vi "Vehicle Control.vi"(11 "stop":bool) -> ()   [LabVIEW 2012]
uses:
  Formula Hybrid 2012 r1/Global Data.vi
  <vilib>/FPGAPlugInAG/cRIO-9076/niLvFpga_Open_cRIO-9076.vi
  <vilib>/rvi/interface/common/dynamic/niFpgaDynamicAddResources.vi
  <vilib>/Utility/error.llb/Error Cluster From Error Code.vi
  <vilib>/rvi/errors/niLvFpgaAdjustHostInterfaceError.vi
  <vilib>/addons/control/pid/pid.llb/PID (DBL).vi
  <vilib>/rvi/interface/nirviOpenFPGA/nirviOpenFPGA.xnode
  FPGA Bitfiles/FormulaHybrid201_FPGATarget_FPGA_E9E2F20A.lvbitx
  Formula Hybrid 2012 r1/FPGA/Sensor Library/FPGA.vi
  <vilib>/rvi/interface/nirviReadWriteControl/nirviReadWriteControl.xnode
  <vilib>/rvi/interface/Simulation/niFpgaSimulationCallBeginRW.vi
  <vilib>/addons/control/pid/NI_PID_pid.lvlib
  NiFpgaLv.dll
panel:
  in  "Lateral PID gains":T1={"proportional gain (Kc)"=1.0, "integral time (Ti, min)"=0.01, "derivative time (Td, min)"=0.0} {"derivative time (Td, min)" format="%.3f"; "integral time (Ti, min)" format="%.3f"; "proportional gain (Kc)" format="%.3f"}
  in  "Allowable Variation from Ideal (Lateral)":dbl=0.1
  in  "Ideal Lateral Slip (%)":dbl=1.2
  out "Throttle Percent":fxp<+,14,1>
  in  "Inline PID gains":T1={"proportional gain (Kc)"=1.0, "integral time (Ti, min)"=0.01, "derivative time (Td, min)"=0.0} {"derivative time (Td, min)" format="%.3f"; "integral time (Ti, min)" format="%.3f"; "proportional gain (Kc)" format="%.3f"}
  in  "Allowable Variation from Ideal (Inline)":dbl=0.1
  in  "Ideal Inline Slip (%)":dbl=1.2
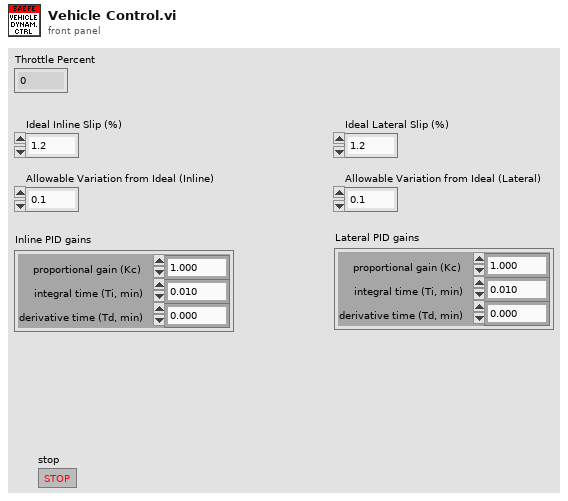
[diagram p1: front panel]
types:
  T1 = cluster{"proportional gain (Kc)":dbl, "integral time (Ti, min)":dbl, "derivative time (Td, min)":dbl}
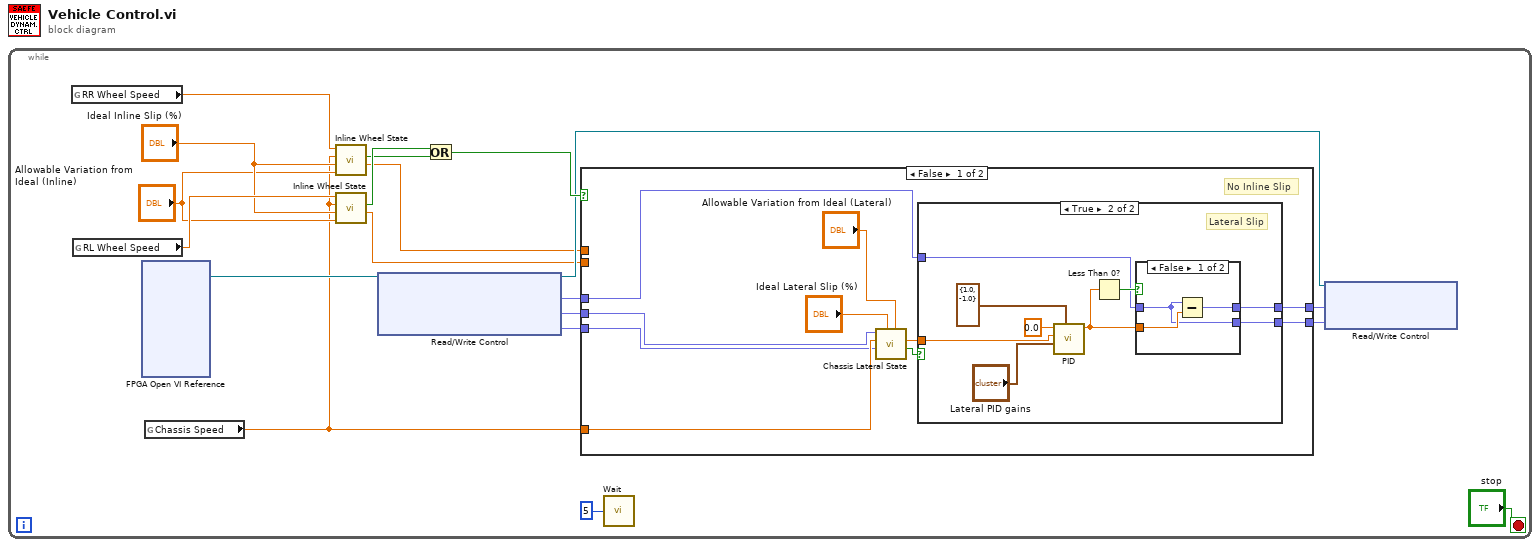
[diagram p0: block diagram]
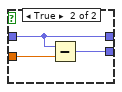
[diagram p3: hidden frame]
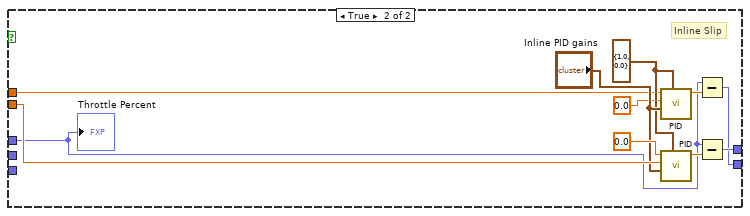
[diagram p4: hidden frame]
diagram:
  n1 = while {
    stop <- "stop" stop-if-true
    n2 = global read "Global Data.vi" "RR Wheel Speed"() -> (w14:dbl)
    n3 = global read "Global Data.vi" "RL Wheel Speed"() -> (w17:dbl)
    n4 = xnode "FPGA Open VI Reference"() -> ("FPGA VI Reference Out"=w10:refnum<k20>)  [unwired: 2 in, 1 out]
    n5 = global read "Global Data.vi" "Chassis Speed"() -> (w3:dbl)
    n6 = call "Inline Wheel State.vi"("Allowable Variation from Ideal"="Allowable Variation from Ideal (Inline)", "Ideal Slip Percent"="Ideal Inline Slip (%)", "Chassis Speed"=w3, "Wheel Speed"=w14) -> ("Error"=w4:dbl, "Inline Slip"=w11:bool)  [unwired: 6 in]
    n7 = call "Inline Wheel State.vi"("Allowable Variation from Ideal"="Allowable Variation from Ideal (Inline)", "Ideal Slip Percent"="Ideal Inline Slip (%)", "Chassis Speed"=w3, "Wheel Speed"=w17) -> ("Error"=w5:dbl, "Inline Slip"=w12:bool)  [unwired: 6 in]
    n8 = xnode "Read/Write Control"("FPGA VI Reference In"=w10) -> ("FPGA VI Reference Out"=w9:refnum<k20>, "Average Throttle (%)"=w8:fxp<+/-,29,18>, "Rotation Rate (degrees/s)"=w2:fxp<+/-,48,26>, "Steering Wheel Angle (degrees)"=w1:fxp<+/-,58,35>)  [unwired: 1 in, 1 out]
    n9 = Or(x=w12, y=w11) -> (x .or. y?=w13:bool)
    n10 = case shown="False" w13 {
      tunnel: w8 -> [w28 w46]
      tunnel: [w27 w53] -> w7
      tunnel: [w26 w47] -> w6
      tunnel: w5 -> [_ w56]
      tunnel: w4 -> [_ w50]
      tunnel: w3 -> [w24 _]
      tunnel: w2 -> [w23 _]
      tunnel: w1 -> [w22 _]
      frame False {
        # "No Inline Slip"
        n11 = call "Chassis Lateral State.vi"("Allowable Variation from Idea"="Allowable Variation from Ideal (Lateral)", "Ideal Lateral Slip"="Ideal Lateral Slip (%)", "Steering Angle"=w22, "Chassis Speed"=w24, "Chassis Yaw Rate"=w23) -> ("Lateral Slip"=w29:bool, "Error"=w25:dbl)  [unwired: 5 in]
        n12 = case shown="True" w29 {
          tunnel: w28 -> [w30 w34]
          tunnel: [w30 w32] -> w27
          tunnel: [w30 w33] -> w26
          tunnel: w25 -> [_ w39]
          frame False {
            # "No Lateral Slip"
          }
          frame True {
            # "Lateral Slip"
            n13 = call-poly <vilib>:"PID.vi"("output range"=cluster{"output high":dbl, "output low":dbl} {"output high"=1.0, "output low"=-1.0}, "PID gains"="Lateral PID gains", "process variable"=w39, "setpoint"=0.0) -> ("output"=w35:dbl)  [unwired: 6 in, 1 out]
            n14 = Less Than 0?(x=w35) -> (x < 0?=w36:bool)
            n15 = case shown="False" w36 {
              tunnel: w35 -> [w42 w45]
              tunnel: w34 -> [w40 w43]
              tunnel: [w40 w44] -> w33
              tunnel: [w41 w43] -> w32
              frame False {
                n16 = Subtract(x=w40, y=w42) -> (x-y=w41:fxp<+,14,1>)
              }
              frame True {
                n17 = Subtract(x=w43, y=w45) -> (x-y=w44:fxp<+,14,1>)
              }
            }
          }
        }
      }
      frame True {
        w51 = cluster{"output high":dbl, "output low":dbl} {"output high"=1.0, "output low"=0.0} ("output range")
        # "Inline Slip"
        n18 = call-poly <vilib>:"PID.vi"("output range"=w51, "PID gains"="Inline PID gains", "process variable"=0.0, "setpoint"=w50) -> ("output"=w48:dbl)  [unwired: 6 in, 1 out]
        n19 = call-poly <vilib>:"PID.vi"("output range"=w51, "PID gains"="Inline PID gains", "process variable"=w56, "setpoint"=0.0) -> ("output"=w54:dbl)  [unwired: 6 in, 1 out]
        n20 = Subtract(x=w46, y=w48) -> (x-y=w47:fxp<+,14,1>)
        n21 = Subtract(x=w46, y=w54) -> (x-y=w53:fxp<+,14,1>)
        "Throttle Percent" <- w46
      }
    }
    n22 = call "Wait"("Count(mSec)"=u32 5) -> ()  [unwired: 1 out]
    n23 = xnode "Read/Write Control"("FPGA VI Reference In"=w9, "Left Throttle Output"=w7, "Right Throttle Output"=w6) -> ()  [unwired: 1 in, 2 out]
  }
